vi "READ_ThorLabs_init.vi"(0 "Init File Name":path=path "C:/LabVIEW_2014/H2O_DIAL/h2o_dial_settings-2.txt", 11 "Error In":errorcluster caption="error in") -> (1 "All Keys Found":bool, 2 "Missing Key Value":bool, 3 "Keys Not Found":string[](array[string]), 4 "Init Keywords and Values":T2(array[cluster]), 6 "ThorLabsCluster":T1, 15 "Error Out":errorcluster)   [LabVIEW 2012]
uses:
  ThorLabsCluster.ctl
  <vilib>/Utility/config.llb/Read Key (Double).vi
  <vilib>/Utility/config.llb/NI_LVConfig.lvlib
panel:
  in  "ThorLabs Init Keys (0-42)":string[](array[string])=["On TEC SLOT", "On LD SLOT", "Off TEC SLOT", "Off LD SLOT", "Etalon TEC SLOT", "TSOA TEC SLOT", "On Temp (C)", "On P-const", "On I-const", "On D-const", "On T-window", "On TempSens", "On Current (mA)", "On Polarity", "On TP-SLOT", "On TP", "Off Temp (C)", "Off P-const", "Off I-const", "Off D-const", "Off T-window", "Off TempSens", "Off Current (mA)", "Off Polarity", "Off TP-SLOT", "Off TP", "Etalon Temp (C)", "Etalon P-const", "Etalon I-const", "Etalon D-const", "Etalon T-window", "Etalon TempSens", "TSOA Temp (C)", "TSOA P-const", "TSOA I-const", "TSOA D-const", "TSOA T-window", "TSOA TempSens", "Warm-up Time (s)", "On Limit (mA)", "On LD Mode", "Off Limit (mA)", "Off LD Mode"]
  # "Read ThorLabs Init"
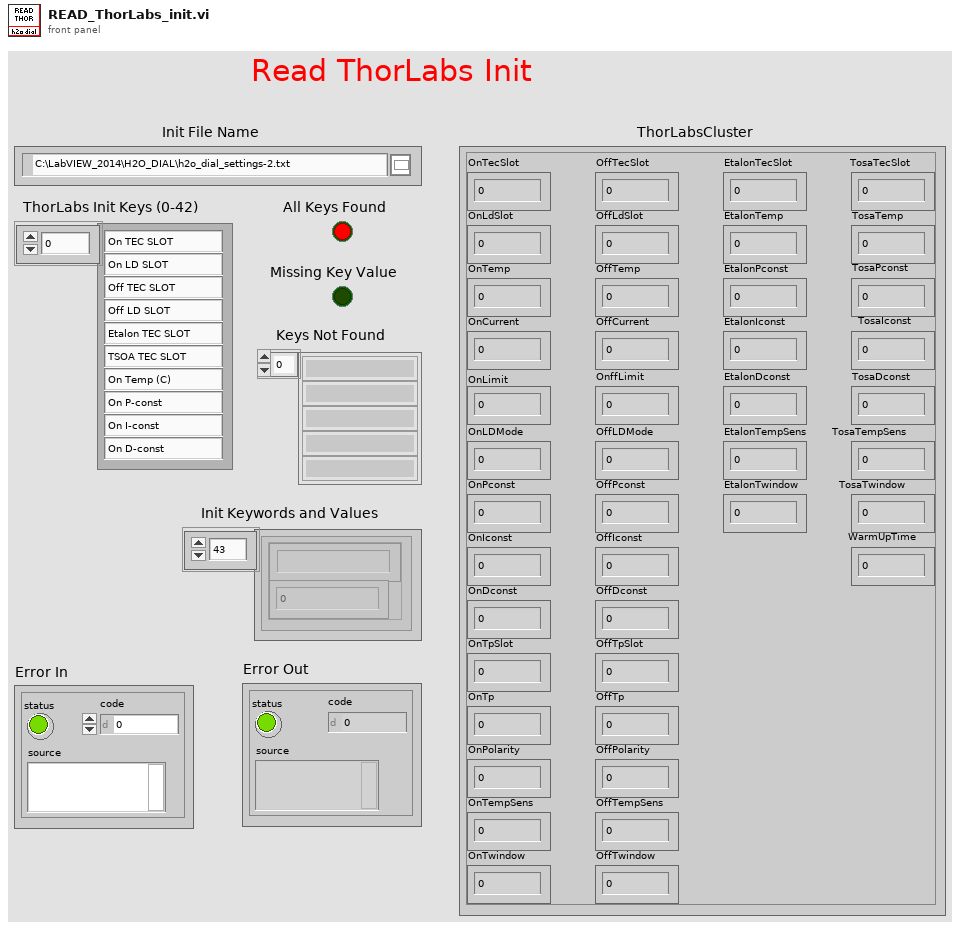
[diagram p1: front panel]
types:
  T1 = typedef "ThorLabsCluster.ctl" = cluster{"OnTecSlot":dbl, "OnLdSlot":dbl, "OnTemp":dbl, "OnCurrent":dbl, "OnLimit":dbl, "OnLDMode":dbl, "OnPconst":dbl, "OnIconst":dbl, "OnDconst":dbl, "OnTpSlot":dbl, "OnTp":dbl, "OnPolarity":dbl, "OnTempSens":dbl, "OnTwindow":dbl, "OffTecSlot":dbl, "OffLdSlot":dbl, "OffTemp":dbl, "OffCurrent":dbl, "OnffLimit":dbl, "OffLDMode":dbl, "OffPconst":dbl, "OffIconst":dbl, "OffDconst":dbl, "OffTpSlot":dbl, "OffTp":dbl, "OffPolarity":dbl, "OffTempSens":dbl, "OffTwindow":dbl, "EtalonTecSlot":dbl, "EtalonTemp":dbl, "EtalonPconst":dbl, "EtalonIconst":dbl, "EtalonDconst":dbl, "EtalonTempSens":dbl, "EtalonTwindow":dbl, "TosaTecSlot":dbl, "TosaTemp":dbl, "TosaPconst":dbl, "TosaIconst":dbl, "TosaDconst":dbl, "TosaTempSens":dbl, "TosaTwindow":dbl, "WarmUpTime":dbl}
  T2 = cluster{"String":string, "Numeric Indicator":dbl}[]
  T3 = typedef "NI_LVConfig.lvlib/Config Data RefNum.ctl" = refnum<k1>
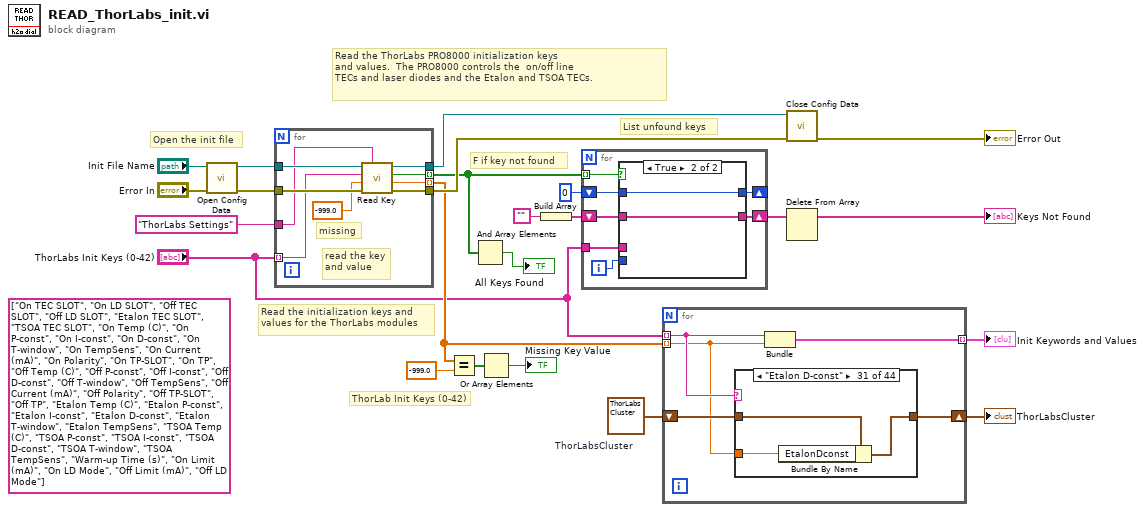
[diagram p0: block diagram]
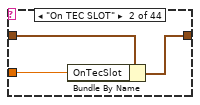
[diagram p3: hidden frame]
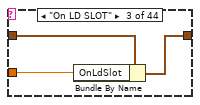
[diagram p4: hidden frame]
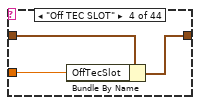
[diagram p5: hidden frame]
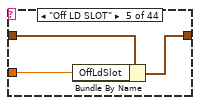
[diagram p6: hidden frame]
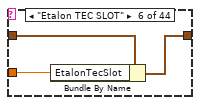
[diagram p7: hidden frame]
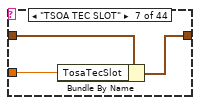
[diagram p8: hidden frame]
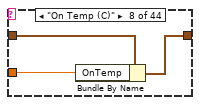
[diagram p9: hidden frame]
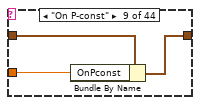
[diagram p10: hidden frame]
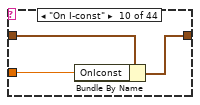
[diagram p11: hidden frame]
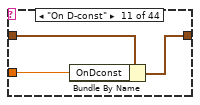
[diagram p12: hidden frame]
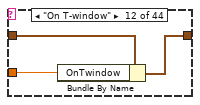
[diagram p13: hidden frame]
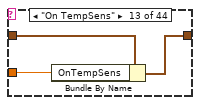
[diagram p14: hidden frame]
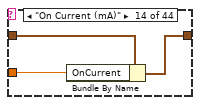
[diagram p15: hidden frame]
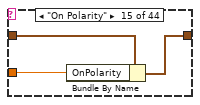
[diagram p16: hidden frame]
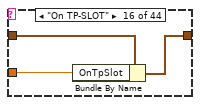
[diagram p17: hidden frame]
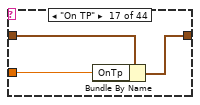
[diagram p18: hidden frame]
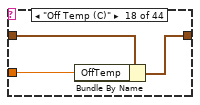
[diagram p19: hidden frame]
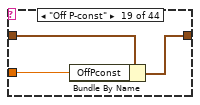
[diagram p20: hidden frame]
diagram:
  w1 = T1 {"OnTecSlot"=0.0, "OnLdSlot"=0.0, "OnTemp"=0.0, "OnCurrent"=0.0, "OnLimit"=0.0, "OnLDMode"=0.0, "OnPconst"=0.0, "OnIconst"=0.0, "OnDconst"=0.0, "OnTpSlot"=0.0, "OnTp"=0.0, "OnPolarity"=0.0, "OnTempSens"=0.0, "OnTwindow"=0.0, "OffTecSlot"=0.0, "OffLdSlot"=0.0, "OffTemp"=0.0, "OffCurrent"=0.0, "OnffLimit"=0.0, "OffLDMode"=0.0, "OffPconst"=0.0, "OffIconst"=0.0, "OffDconst"=0.0, "OffTpSlot"=0.0, "OffTp"=0.0, "OffPolarity"=0.0, "OffTempSens"=0.0, "OffTwindow"=0.0, "EtalonTecSlot"=0.0, "EtalonTemp"=0.0, "EtalonPconst"=0.0, "EtalonIconst"=0.0, "EtalonDconst"=0.0, "EtalonTempSens"=0.0, "EtalonTwindow"=0.0, "TosaTecSlot"=0.0, "TosaTemp"=0.0, "TosaPconst"=0.0, "TosaIconst"=0.0, "TosaDconst"=0.0, "TosaTempSens"=0.0, "TosaTwindow"=0.0, "WarmUpTime"=0.0}  # ThorLabsCluster
  (unwired) string[] ["On TEC SLOT", "On LD SLOT", "Off TEC SLOT", "Off LD SLOT", "Etalon TEC SLOT", "TSOA TEC SLOT", "On Temp (C)", "On P-const", "On I-const", "On D-const", "On T-window", "On TempSens", "On Current (mA)", "On Polarity", "On TP-SLOT", "On TP", "Off Temp (C)", "Off P-const", "Off I-const", "Off D-const", "Off T-window", "Off TempSens", "Off Current (mA)", "Off Polarity", "Off TP-SLOT", "Off TP", "Etalon Temp (C)", "Etalon P-const", "Etalon I-const", "Etalon D-const", "Etalon T-window", "Etalon TempSens", "TSOA Temp (C)", "TSOA P-const", "TSOA I-const", "TSOA D-const", "TSOA T-window", "TSOA TempSens", "Warm-up Time (s)", "On Limit (mA)", "On LD Mode", "Off Limit (mA)", "Off LD Mode"] ("ThorLabs Init Keys (0-42) 2")
  # "ThorLab Init Keys (0-42)"
  # "F if key not found"
  # "Open the init file"
  # "List unfound keys"
  # "Read the initialization keys and\nvalues for the ThorLabs modules"
  # "Read the ThorLabs PRO8000 initialization keys\nand values.  The PRO8000 controls the  on/off line\nTECs and laser diodes and the Etalon and TSOA TECs."
  n1 = call <vilib>:"Open Config Data.vi"("error in (no error)"="Error In", "configuration file path"="Init File Name") -> ("error out"=w21:errorcluster, "refnum"=w20:T3)  [unwired: 1 in, 7 out]
  n2 = for {
    tunnel: w21 -> [w31]
    tunnel: w20 -> [w32]
    tunnel: "ThorLabs Init Keys (0-42)" -> [w30] mode=indexing
    tunnel: "ThorLabs Settings" ("section") -> [w25]
    tunnel: [w29] -> w5 mode=indexing
    tunnel: [w28] -> w10 mode=indexing
    tunnel: [w27] -> w18
    tunnel: [w26] -> w17
    # "missing"
    # "read the key\nand value"
    n3 = call-poly <vilib>:"Read Key.vi"("section"=w25, "error in (no error)"=w31, "default value"=-999.0, "key"=w30, "refnum"=w32) -> ("error out"=w26:errorcluster, "value"=w29:dbl, "found?"=w28:bool, "refnum out"=w27:T3)  [unwired: 3 in]
  }
  n4 = Equal?(x=w5, y=-999.0) -> (x = y?=w7:bool[])
  n5 = And Array Elements(Boolean array=w10) -> (logical AND=→"All Keys Found":bool)
  n6 = Or Array Elements(Boolean array=w7) -> (logical OR=→"Missing Key Value":bool)
  n7 = Build Array("") -> (w14:string[])
  n8 = for {
    tunnel: w10 -> [w38] mode=indexing
    shift-right: [w39] -> _
    shift-left: 0 -> [w36]
    shift-right: [w35] -> w11
    shift-left: w14 -> [w37]
    tunnel: "ThorLabs Init Keys (0-42)" -> [w34]
    i -> [w33]
    n9 = case shown="True" w38 {
      tunnel: w36 -> [w41 w48]
      tunnel: [w46 w48] -> w39
      tunnel: w33 -> [w44 _]
      tunnel: w37 -> [w45 w47]
      tunnel: [w42 w47] -> w35
      tunnel: w34 -> [w43 _]
      frame False {
        n10 = Increment(x=w41) -> (x+1=w46:i32)
        n11 = Index Array(array=w43, index=w44) -> (element=w40:string)
        n12 = Insert Into Array(array=w45, index=w41, new element=w40) -> (w42:string[])
      }
      frame True {
      }
    }
  }
  n13 = for {
    tunnel: "ThorLabs Init Keys (0-42)" -> [w50] mode=indexing
    tunnel: w5 -> [w49] mode=indexing
    tunnel: [w53] -> w4 mode=indexing
    shift-right: [w51] -> w2
    shift-left: w1 -> [w52]
    n14 = case shown="\"Etalon D-const\"" w50 {
      tunnel: w52 -> [w54 w56 w59 w62 w65 w68 w71 w74 w77 w80 w83 w86 w89 w92 w95 w98 w101 w104 w107 w110 w113 w116 w119 w122 w125 w128 w131 w134 w137 w140 w143 w146 w149 w152 w155 w158 w161 w164 w167 w170 w173 w176 w179 w182]
      tunnel: [w54 w55 w58 w61 w64 w67 w70 w73 w76 w79 w82 w85 w88 w91 w94 w97 w100 w103 w106 w109 w112 w115 w118 w121 w124 w127 w130 w133 w136 w139 w142 w145 w148 w151 w154 w157 w160 w163 w166 w169 w172 w175 w178 w181] -> w51
      tunnel: w49 -> [_ w57 w60 w63 w66 w69 w72 w75 w78 w81 w84 w87 w90 w93 w96 w99 w102 w105 w108 w111 w114 w117 w120 w123 w126 w129 w132 w135 w138 w141 w144 w147 w150 w153 w156 w159 w162 w165 w168 w171 w174 w177 w180 w183]
      frame Default {
      }
      frame "On TEC SLOT" {
        n15 = Bundle By Name(cluster=w56, "OnTecSlot"=w57) -> (w55:T1)
      }
      frame "On LD SLOT" {
        n16 = Bundle By Name(cluster=w59, "OnLdSlot"=w60) -> (w58:T1)
      }
      frame "Off TEC SLOT" {
        n17 = Bundle By Name(cluster=w62, "OffTecSlot"=w63) -> (w61:T1)
      }
      frame "Off LD SLOT" {
        n18 = Bundle By Name(cluster=w65, "OffLdSlot"=w66) -> (w64:T1)
      }
      frame "Etalon TEC SLOT" {
        n19 = Bundle By Name(cluster=w68, "EtalonTecSlot"=w69) -> (w67:T1)
      }
      frame "TSOA TEC SLOT" {
        n20 = Bundle By Name(cluster=w71, "TosaTecSlot"=w72) -> (w70:T1)
      }
      frame "On Temp (C)" {
        n21 = Bundle By Name(cluster=w74, "OnTemp"=w75) -> (w73:T1)
      }
      frame "On P-const" {
        n22 = Bundle By Name(cluster=w77, "OnPconst"=w78) -> (w76:T1)
      }
      frame "On I-const" {
        n23 = Bundle By Name(cluster=w80, "OnIconst"=w81) -> (w79:T1)
      }
      frame "On D-const" {
        n24 = Bundle By Name(cluster=w83, "OnDconst"=w84) -> (w82:T1)
      }
      frame "On T-window" {
        n25 = Bundle By Name(cluster=w86, "OnTwindow"=w87) -> (w85:T1)
      }
      frame "On TempSens" {
        n26 = Bundle By Name(cluster=w89, "OnTempSens"=w90) -> (w88:T1)
      }
      frame "On Current (mA)" {
        n27 = Bundle By Name(cluster=w92, "OnCurrent"=w93) -> (w91:T1)
      }
      frame "On Polarity" {
        n28 = Bundle By Name(cluster=w95, "OnPolarity"=w96) -> (w94:T1)
      }
      frame "On TP-SLOT" {
        n29 = Bundle By Name(cluster=w98, "OnTpSlot"=w99) -> (w97:T1)
      }
      frame "On TP" {
        n30 = Bundle By Name(cluster=w101, "OnTp"=w102) -> (w100:T1)
      }
      frame "Off Temp (C)" {
        n31 = Bundle By Name(cluster=w104, "OffTemp"=w105) -> (w103:T1)
      }
      frame "Off P-const" {
        n32 = Bundle By Name(cluster=w107, "OffPconst"=w108) -> (w106:T1)
      }
      frame "Off I-const" {
        n33 = Bundle By Name(cluster=w110, "OffIconst"=w111) -> (w109:T1)
      }
      frame "Off D-const" {
        n34 = Bundle By Name(cluster=w113, "OffDconst"=w114) -> (w112:T1)
      }
      frame "Off T-window" {
        n35 = Bundle By Name(cluster=w116, "OffTwindow"=w117) -> (w115:T1)
      }
      frame "Off TempSens" {
        n36 = Bundle By Name(cluster=w119, "OffTempSens"=w120) -> (w118:T1)
      }
      frame "Off Current (mA)" {
        n37 = Bundle By Name(cluster=w122, "OffCurrent"=w123) -> (w121:T1)
      }
      frame "Off Polarity" {
        n38 = Bundle By Name(cluster=w125, "OffPolarity"=w126) -> (w124:T1)
      }
      frame "Off TP-SLOT" {
        n39 = Bundle By Name(cluster=w128, "OffTpSlot"=w129) -> (w127:T1)
      }
      frame "Off TP" {
        n40 = Bundle By Name(cluster=w131, "OffTp"=w132) -> (w130:T1)
      }
      frame "Etalon Temp (C)" {
        n41 = Bundle By Name(cluster=w134, "EtalonTemp"=w135) -> (w133:T1)
      }
      frame "Etalon P-const" {
        n42 = Bundle By Name(cluster=w137, "EtalonPconst"=w138) -> (w136:T1)
      }
      frame "Etalon I-const" {
        n43 = Bundle By Name(cluster=w140, "EtalonIconst"=w141) -> (w139:T1)
      }
      frame "Etalon D-const" {
        n44 = Bundle By Name(cluster=w143, "EtalonDconst"=w144) -> (w142:T1)
      }
      frame "Etalon T-window" {
        n45 = Bundle By Name(cluster=w146, "EtalonTwindow"=w147) -> (w145:T1)
      }
      frame "Etalon TempSens" {
        n46 = Bundle By Name(cluster=w149, "EtalonTempSens"=w150) -> (w148:T1)
      }
      frame "TSOA Temp (C)" {
        n47 = Bundle By Name(cluster=w152, "TosaTemp"=w153) -> (w151:T1)
      }
      frame "TSOA P-const" {
        n48 = Bundle By Name(cluster=w155, "TosaPconst"=w156) -> (w154:T1)
      }
      frame "TSOA I-const" {
        n49 = Bundle By Name(cluster=w158, "TosaIconst"=w159) -> (w157:T1)
      }
      frame "TSOA D-const" {
        n50 = Bundle By Name(cluster=w161, "TosaDconst"=w162) -> (w160:T1)
      }
      frame "TSOA T-window" {
        n51 = Bundle By Name(cluster=w164, "TosaTwindow"=w165) -> (w163:T1)
      }
      frame "TSOA TempSens" {
        n52 = Bundle By Name(cluster=w167, "TosaTempSens"=w168) -> (w166:T1)
      }
      frame "Warm-up Time (s)" {
        n53 = Bundle By Name(cluster=w170, "WarmUpTime"=w171) -> (w169:T1)
      }
      frame "On Limit (mA)" {
        n54 = Bundle By Name(cluster=w173, "OnLimit"=w174) -> (w172:T1)
      }
      frame "On LD Mode" {
        n55 = Bundle By Name(cluster=w176, "OnLDMode"=w177) -> (w175:T1)
      }
      frame "Off Limit (mA)" {
        n56 = Bundle By Name(cluster=w179, "OnffLimit"=w180) -> (w178:T1)
      }
      frame "Off LD Mode" {
        n57 = Bundle By Name(cluster=w182, "OffLDMode"=w183) -> (w181:T1)
      }
    }
    n58 = Bundle("String"=w50, "value"=w49) -> (w53:cluster{"String":string, "value":dbl})  [unwired: 1 in]
  }
  "Init Keywords and Values" <- w4
  "ThorLabsCluster" <- w2
  n59 = call <vilib>:"Close Config Data.vi"("error in (no error)"=w17, "refnum"=w18) -> ("error out"=→"Error Out":errorcluster)  [unwired: 1 in, 8 out]
  n60 = Delete From Array(array=w11) -> (array with subset deleted=→"Keys Not Found":string[])  [unwired: 2 in, 1 out]
